vi "close_memtest_N_v02.vi"(4 "which clamp":enum16{"VClamp", "IClamp"}(ring), 6 "memtest":T1={"Samples to Read"=1000, "Rate (Hz)"=20000.0, "Amplitude (mV/pA)"=10.0, "Offset (mV/pA)"=-60.0, "Frequency (Hz)"=-60.0, "duty cycle (%)"=50.0, "phase"=0.0} {"phase" format="%.2p"; "duty cycle (%)" format="%0.2f"}, 7 "AO physical channels":tag="cDAQ1Mod3/ao14", 8 "AI error in":errorcluster, 9 "AO task in":refnum<k21>, 10 "AO error in":errorcluster, 11 "AI task in":refnum<k21>) -> (0 "error out":errorcluster)   [LabVIEW 2015]
uses:
  <vilib>/DAQmx/create/channels.llb/DAQmx Create Channel (AO-Voltage-Basic).vi
  <vilib>/DAQmx/write.llb/DAQmx Write (Analog 1D DBL NChan 1Samp).vi
  <resource>/objmgr/daqmx.rc
  controls/memtest_def.ctl
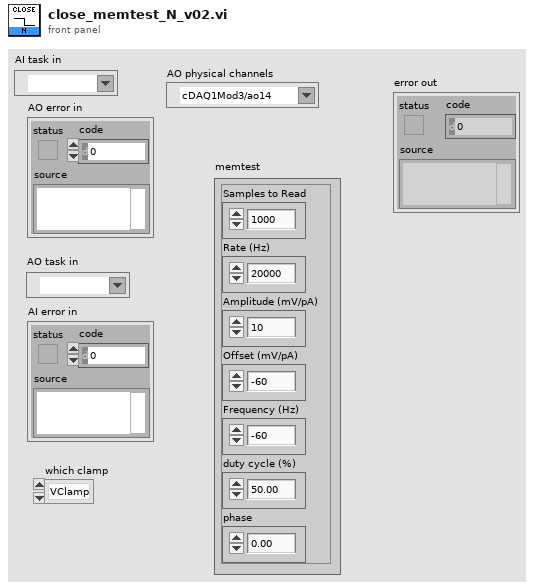
[diagram p1: front panel]
types:
  T1 = typedef "memtest_def.ctl" = cluster{"Samples to Read":i32, "Rate (Hz)":dbl, "Amplitude (mV/pA)":dbl, "Offset (mV/pA)":dbl, "Frequency (Hz)":dbl, "duty cycle (%)":dbl, "phase":dbl}
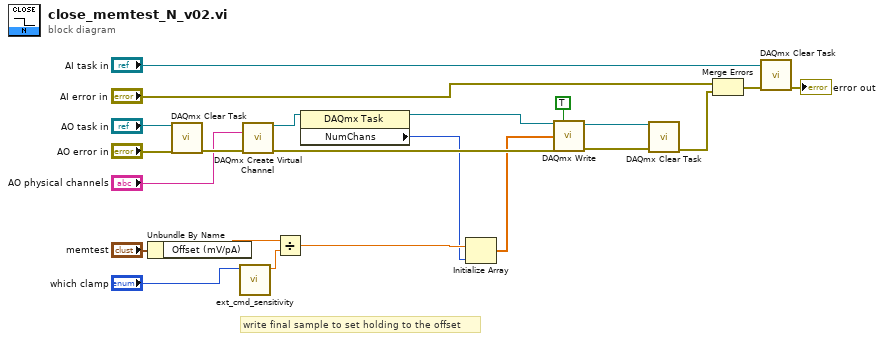
[diagram p0: block diagram]
diagram:
  # "write final sample to set holding to the offset"
  n1 = Unbundle By Name("memtest") -> ("Offset (mV/pA)"=w9:dbl)
  n2 = call <vilib>:"DAQmx Clear Task.vi"("task in"="AO task in", "error in"="AO error in") -> ("error out"=w20:errorcluster)  [unwired: 13 in]
  n3 = call "ext_cmd_sensitivity.vi"("which clamp"="which clamp") -> ("division factor"=w6:dbl)  [unwired: 10 in]
  n4 = call-poly <vilib>:"DAQmx Create Virtual Channel.vi"("physical channels"="AO physical channels", "error in"=w20) -> ("task out"=w5:refnum<k21>, "error out"=w17:errorcluster)  [unwired: 12 in]
  n5 = Divide(x=w9, y=w6) -> (x/y=w3:dbl)
  n6 = property class="DAQmx Task"(reference=w5) -> (reference out=w4:refnum<k21>, "NumChans"=w2:u32)  [unwired: 1 in, 1 out]
  n7 = Initialize Array(w3, w2) -> (w1:dbl[])
  n8 = call-poly <vilib>:"DAQmx Write.vi"("task/channels in"=w4, "auto start"=TRUE, "data"=w1, "error in"=w17) -> ("task out"=w16:refnum<k21>, "error out"=w15:errorcluster)  [unwired: 9 in, 1 out]
  n9 = call <vilib>:"DAQmx Clear Task.vi"("task in"=w16, "error in"=w15) -> ("error out"=w12:errorcluster)  [unwired: 13 in]
  n10 = Merge Errors("AI error in", w12) -> (w13:errorcluster)
  n11 = call <vilib>:"DAQmx Clear Task.vi"("task in"="AI task in", "error in"=w13) -> ("error out"=→"error out":errorcluster)  [unwired: 13 in]
